vi "Open IMAQ IO.vi"   [LabVIEW 2013]
doc: "Opens a reference to your IMAQ I/O device."
uses:
  <vilib>/FPGAPlugInAG/IMAQIO-5/niLvFpga_Open_IMAQIO-5.vi
  <vilib>/rvi/interface/nirviOpenFPGA/nirviOpenFPGA.xnode
  <vilib>/LabVIEW Targets/FPGA/IMAQIO/Default IMAQIO (FPGA).lvbitx
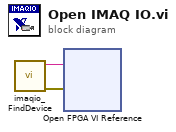
[diagram p0: block diagram]
diagram:
  n1 = call <vilib>:"imaqio_FindDevice.vi"() -> ("error out"=w2:errorcluster, "Resource Out"=w1:string)  [unwired: 2 in, 8 out]
  n2 = xnode "Open FPGA VI Reference"("error in"=w2, "resource name"=w1) -> ()  [unwired: 2 out]
